vi "Frame convert.vi"(10 "Frame":string[](array[string])) -> (2 "ID":u32, 3 "CAN frame":T1 {"payload" format="%x"; "timestamp" format="%<%.7X\n%x>T"; "type" items=["CAN Data"=0, "CAN Remote"=1, "CAN Bus Error"=2, "CAN 2.0 Data"=8, "CAN FD Data"=16, "CAN FD+BRS Data"=24, "J1939 Data"=192, "Delay"=224, "Log Trigger"=225, "Start Trigger"=226]; "identifier" format="%x"})   [LabVIEW 2025, in "CAN-LIN Raw Bus Capture UI.lvlib"]
uses:
  CAN-LIN Raw Bus Capture UI.lvlib
  <vilib>/xnet/xnet.llb/XNET Frame CAN.ctl
  <vilib>/xnet/xnet.llb/XNET Frame Type CAN.ctl
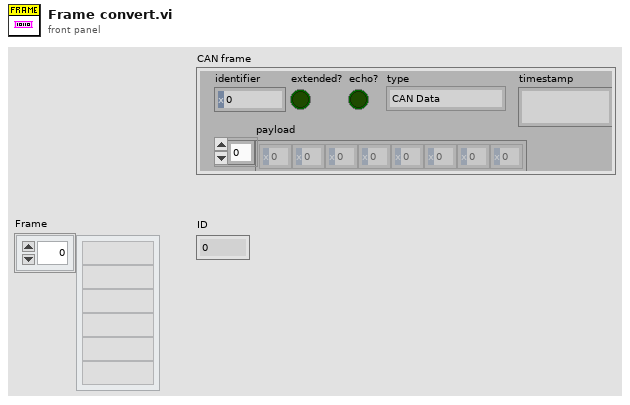
[diagram p1: front panel]
types:
  T1 = typedef "XNET Frame CAN.ctl" = cluster{"timestamp":timestamp, "payload":u8[], "identifier":u32, "type":T2, "extended?":bool, "echo?":bool}
  T2 = typedef "XNET Frame Type CAN.ctl" = u8
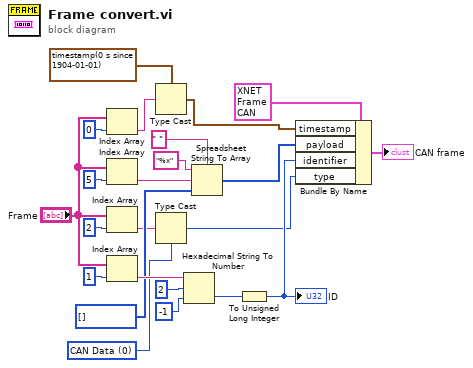
[diagram p0: block diagram]
diagram:
  w3 = T2 0 items=["CAN Data"=0, "CAN Remote"=1, "CAN Bus Error"=2, "CAN 2.0 Data"=8, "CAN FD Data"=16, "CAN FD+BRS Data"=24, "J1939 Data"=192, "Delay"=224, "Log Trigger"=225, "Start Trigger"=226] ("type")
  n1 = Index Array(array="Frame", index=0) -> (element=w12:string)
  n2 = Index Array(array="Frame", index=5) -> (element=w9:string)
  n3 = Index Array(array="Frame", index=2) -> (element=w2:string)
  n4 = Index Array(array="Frame", index=1) -> (element=w18:string)
  n5 = Type Cast(type=timestamp(0 s since 1904-01-01) ("timestamp"), x=w12) -> (*(type *) &x=w22:timestamp)
  n6 = Type Cast(type=w3, x=w2) -> (*(type *) &x=w1:T2)
  n7 = Hexadecimal String To Number(string=w18, offset=2, default (0uL)=-1 ("default (0 U32)")) -> (number=w15:i32)  [unwired: 1 out]
  n8 = Spreadsheet String To Array(delimiter (Tab)=" ", format string="%x", spreadsheet string=w9, array type (2D Dbl)=u8[] [] ("payload")) -> (array=w6:u8[])
  n9 = To Unsigned Long Integer(number=w15) -> (unsigned 32bit integer=w14:u32)
  "ID" <- w14
  n10 = Bundle By Name(cluster=T1 {"timestamp"=timestamp(0 s since 1904-01-01), "payload"=[50, 32, 3, 0, 0], "identifier"=291, "type"=0, "extended?"=FALSE, "echo?"=FALSE} ("CAN frame"), "timestamp"=w22, "payload"=w6, "identifier"=w14, "type"=w1) -> (→"CAN frame":T1)
